vi "main.vi"() -> ()   [LabVIEW 2023] (continued)
  8        F0\t60\t22\tFC\tFF\tFF\tFF\t43\r\n      1144  0CF103A7   00000004    8        17\t1F\t08\t60\tB1\t1F\t08\t43\r\n      1144  0CF102A7   00000004    8        30\t75\tE0\t2E\t80\tFF\tFF\tFD\r\n      1143  0C3C4D4A   00000004    8        BE\tFF\tFF\t7F\t18\tFF\tFF\t43\r\n      1143  0CF101A7   00000004    8        68\t00\t97\tCC\t00\t15\t39\t53\r\n      1142  18F120F0   00000004    8        2B\t75\t60\tB1\tB0\t01\tFF\tFF\r\n      1141  18F11FF0   00000004    8        FF\t3F\t90\t68\t88\t1B\t10\t3C\r\n      1132  1FFFFFFF   00000004    8        00\t20\tFF\tFF\tFF\tFF\tFF\tFF\r\n      1147  18FEF117   00000004    8        F7\t97\tCC\tCF\tFF\tFF\tFF\tFF\r\n      1147  18F121F0   00000004    8        09\t18\t00\t00\tFF\tFF\tB0\t01\r\n      1146  18F108A7   00000004    8        F0\t00\t00\tFF\tFF\tFF\tFF\t40\r\n      1145  18F106A7   00000004    8        00\tF7\tFF\tFF\tFF\tFF\tFF\t87\r\n      1145  0CF104A7   00000004    8        F0\t60\t22\tFC\tFF\tFF\tFF\t43\r\n      1144  0CF103A7   00000004    8        17\t1F\t08\t60\tB1\t1F\t08\t43\r\n      1144  0CF102A7   00000004    8        30\t75\tE0\t2E\t80\tFF\tFF\tFD\r\n      1143  0C3C4D4A   00000004    8        BE\tFF\tFF\t7F\t18\tFF\tFF\t43\r\n      1143  0CF101A7   00000004    8        68\t00\t97\tCC\t00\t15\t39\t53\r\n      1142  18F120F0   00000004    8        2B\t75\t60\tB1\tB0\t01\tFF\tFF\r\n      1141  18F11FF0   00000004    8        FF\t3F\t90\t68\t88\t1B\t10\t3C\r\n      1148  1FFFFFFF   00000004    8        00\t00\tFF\tFF\tFF\tFF\tFF\tFF\r\n      1147  18FEF117   00000004    8        F7\t97\tCC\tCF\tFF\tFF\tFF\tFF\r\n      1147  18F121F0   00000004    8        09\t18\t00\t00\tFF\tFF\tB0\t01\r\n      1146  18F108A7   00000004    8        F0\t00\t00\tFF\tFF\tFF\tFF\t40\r\n      1145  18F106A7   00000004    8        00\tF7\tFF\tFF\tFF\tFF\tFF\t87\r\n      1145  0CF104A7   00000004    8        F0\t60\t22\tFC\tFF\tFF\tFF\t43\r\n      1144  0CF103A7   00000004    8        17\t1F\t08\t60\tB1\t1F\t08\t43\r\n      1144  0CF102A7   00000004    8        30\t75\tE0\t2E\t80\tFF\tFF\tFD\r\n      1143  0C3C4D4A   00000004    8        BE\tFF\tFF\t7F\t18\tFF\tFF\t43\r\n      1143  0CF101A7   00000004    8        68\t00\t97\tCC\t00\t15\t39\t53\r\n      1142  18F120F0   00000004    8        2B\t75\t60\tB1\tB0\t01\tFF\tFF\r\n      1152  1FFFFFFF   00000004    8        00\t20\tFF\tFF\tFF\tFF\tFF\tFF\r\n      1148  1FFFFFFF   00000004    8        00\t00\tFF\tFF\tFF\tFF\tFF\tFF\r\n      1147  18FEF117   00000004    8        F7\t97\tCC\tCF\tFF\tFF\tFF\tFF\r\n      1147  18F121F0   00000004    8        09\t18\t00\t00\tFF\tFF\tB0\t01\r\n      1146  18F108A7   00000004    8        F0\t00\t00\tFF\tFF\tFF\tFF\t40\r\n      1145  18F106A7   00000004    8        00\tF7\tFF\tFF\tFF\tFF\tFF\t87\r\n      1145  0CF104A7   00000004    8        F0\t60\t22\tFC\tFF\tFF\tFF\t43\r\n      1144  0CF103A7   00000004    8        17\t1F\t08\t60\tB1\t1F\t08\t43\r\n      1144  0CF102A7   00000004    8        30\t75\tE0\t2E\t80\tFF\tFF\tFD\r\n      1143  0C3C4D4A   00000004    8        BE\tFF\tFF\t7F\t18\tFF\tFF\t43\r\n      1143  0CF101A7   00000004    8        68\t00\t97\tCC\t00\t15\t39\t53\r\n      1162  1FFFFFFF   00000004    8        00\t20\tFF\tFF\tFF\tFF\tFF\tFF\r\n      1152  1FFFFFFF   00000004    8        00\t20\tFF\tFF\tFF\tFF\tFF\tFF\r\n      1148  1FFFFFFF   00000004    8        00\t00\tFF\tFF\tFF\tFF\tFF\tFF\r\n      1147  18FEF117   00000004    8        F7\t97\tCC\tCF\tFF\tFF\tFF\tFF\r\n      1147  18F121F0   00000004    8        09\t18\t00\t00\tFF\tFF\tB0\t01\r\n      1146  18F108A7   00000004    8        F0\t00\t00\tFF\tFF\tFF\tFF\t40\r\n      1145  18F106A7   00000004    8        00\tF7\tFF\tFF\tFF\tFF\tFF\t87\r\n      1145  0CF104A7   00000004    8        F0\t60\t22\tFC\tFF\tFF\tFF\t43\r\n      1144  0CF103A7   00000004    8        17\t1F\t08\t60\tB1\t1F\t08\t43\r\n      1144  0CF102A7   00000004    8        30\t75\tE0\t2E\t80\tFF\tFF\tFD\r\n      1143  0C3C4D4A   00000004    8        BE\tFF\tFF\t7F\t18\tFF\tFF\t43\r\n      1163  0CF101A7   00000004    8        68\t00\t97\tCC\t00\t15\t39\t54\r\n      1162  1FFFFFFF   00000004    8        00\t20\tFF\tFF\tFF\tFF\tFF\tFF\r\n      1152  1FFFFFFF   00000004    8        00\t20\tFF\tFF\tFF\tFF\tFF\tFF\r\n      1148  1FFFFFFF   00000004    8        00\t00\tFF\tFF\tFF\tFF\tFF\tFF\r\n      1147  18FEF117   00000004    8        F7\t97\tCC\tCF\tFF\tFF\tFF\tFF\r\n      1147  18F121F0   00000004    8        09\t18\t00\t00\tFF\tFF\tB0\t01\r\n      1146  18F108A7   00000004    8        F0\t00\t00\tFF\tFF\tFF\tFF\t40\r\n      1145  18F106A7   00000004    8        00\tF7\tFF\tFF\tFF\tFF\tFF\t87\r\n      1145  0CF104A7   00000004    8        F0\t60\t22\tFC\tFF\tFF\tFF\t43\r\n      1144  0CF103A7   00000004    8        17\t1F\t08\t60\tB1\t1F\t08\t43\r\n      1144  0CF102A7   00000004    8        30\t75\tE0\t2E\t80\tFF\tFF\tFD\r\n      1163  0CF102A7   00000004    8        30\t75\tE0\t2E\t80\tFF\tFF\tFD\r\n      1163  0CF101A7   00000004    8        68\t00\t97\tCC\t00\t15\t39\t54\r\n      1162  1FFFFFFF   00000004    8        00\t20\tFF\tFF\tFF\tFF\tFF\tFF\r\n      1152  1FFFFFFF   00000004    8        00\t20\tFF\tFF\tFF\tFF\tFF\tFF\r\n      1148  1FFFFFFF   00000004    8        00\t00\tFF\tFF\tFF\tFF\tFF\tFF\r\n      1147  18FEF117   00000004    8        F7\t97\tCC\tCF\tFF\tFF\tFF\tFF\r\n      1147  18F121F0   00000004    8        09\t18\t00\t00\tFF\tFF\tB0\t01\r\n      1146  18F108A7   00000004    8        F0\t00\t00\tFF\tFF\tFF\tFF\t40\r\n      1145  18F106A7   00000004    8        00\tF7\tFF\tFF\tFF\tFF\tFF\t87\r\n      1145  0CF104A7   00000004    8        F0\t60\t22\tFC\tFF\tFF\tFF\t43\r\n      1144  0CF103A7   00000004    8        17\t1F\t08\t60\tB1\t1F\t08\t43\r\n      1172  1FFFFFFF   00000004    8        00\t20\tFF\tFF\tFF\tFF\tFF\tFF\r\n      1163  0CF102A7   00000004    8        30\t75\tE0\t2E\t80\tFF\tFF\tFD\r\n      1163  0CF101A7   00000004    8        68\t00\t97\tCC\t00\t15\t39\t54\r\n      1162  1FFFFFFF   00000004    8        00\t20\tFF\tFF\tFF\tFF\tFF\tFF\r\n      1152  1FFFFFFF   00000004    8        00\t20\tFF\tFF\tFF\tFF\tFF\tFF\r\n      1148  1FFFFFFF   00000004    8        00\t00\tFF\tFF\tFF\tFF\tFF\tFF\r\n      1147  18FEF117   00000004    8        F7\t97\tCC\tCF\tFF\tFF\tFF\tFF\r\n      1147  18F121F0   00000004    8        09\t18\t00\t00\tFF\tFF\tB0\t01\r\n      1146  18F108A7   00000004    8        F0\t00\t00\tFF\tFF\tFF\tFF\t40\r\n      1145  18F106A7   00000004    8        00\tF7\tFF\tFF\tFF\tFF\tFF\t87\r\n      1145  0CF104A7   00000004    8        F0\t60\t22\tFC\tFF\tFF\tFF\t43\r\n      1182  1FFFFFFF   00000004    8        00\t00\tFF\tFF\tFF\tFF\tFF\tFF\r\n      1172  1FFFFFFF   00000004    8        00\t20\tFF\tFF\tFF\tFF\tFF\tFF\r\n      1163  0CF102A7   00000004    8        30\t75\tE0\t2E\t80\tFF\tFF\tFD\r\n      1163  0CF101A7   00000004    8        68\t00\t97\tCC\t00\t15\t39\t54\r\n      1162  1FFFFFFF   00000004    8        00\t20\tFF\tFF\tFF\tFF\tFF\tFF\r\n      1152  1FFFFFFF   00000004    8        00\t20\tFF\tFF\tFF\tFF\tFF\tFF\r\n      1148  1FFFFFFF   00000004    8        00\t00\tFF\tFF\tFF\tFF\tFF\tFF\r\n      1147  18FEF117   00000004    8        F7\t97\tCC\tCF\tFF\tFF\tFF\tFF\r\n      1147  18F121F0   00000004    8        09\t18\t00\t00\tFF\tFF\tB0\t01\r\n      1146  18F108A7   00000004    8        F0\t00\t00\tFF\tFF\tFF\tFF\t40\r\n      1145  18F106A7   00000004    8        00\tF7\tFF\tFF\tFF\tFF\tFF\t87\r\n      1183  0CF101A7   00000004    8        68\t00\t97\tCC\t00\t15\t39\t55\r\n      1182  1FFFFFFF   00000004    8        00\t00\tFF\tFF\tFF\tFF\tFF\tFF\r\n      1172  1FFFFFFF   00000004    8        00\t20\tFF\tFF\tFF\tFF\tFF\tFF\r\n      1163  0CF102A7   00000004    8        30\t75\tE0\t2E\t80\tFF\tFF\tFD\r\n      1163  0CF101A7   00000004    8        68\t00\t97\tCC\t00\t15\t39\t54\r\n      1162  1FFFFFFF   00000004    8        00\t20\tFF\tFF\tFF\tFF\tFF\tFF\r\n      1152  1FFFFFFF   00000004    8        00\t20\tFF\tFF\tFF\tFF\tFF\tFF\r\n      1148  1FFFFFFF   00000004    8        00\t00\tFF\tFF\tFF\tFF\tFF\tFF\r\n      1147  18FEF117   00000004    8        F7\t97\tCC\tCF\tFF\tFF\tFF\tFF\r\n      1147  18F121F0   00000004    8        09\t18\t00\t00\tFF\tFF\tB0\t01\r\n      1146  18F108A7   00000004    8        F0\t00\t00\tFF\tFF\tFF\tFF\t40\r\n      1183  0CF102A7   00000004    8        30\t75\tE0\t2E\t80\tFF\tFF\tFD\r\n      1183  0CF101A7   00000004    8        68\t00\t97\tCC\t00\t15\t39\t55\r\n      1182  1FFFFFFF   00000004    8        00\t00\tFF\tFF\tFF\tFF\tFF\tFF\r\n      1172  1FFFFFFF   00000004    8        00\t20\tFF\tFF\tFF\tFF\tFF\tFF\r\n      1163  0CF102A7   00000004    8        30\t75\tE0\t2E\t80\tFF\tFF\tFD\r\n      1163  0CF101A7   00000004    8        68\t00\t97\tCC\t00\t15\t39\t54\r\n      1162  1FFFFFFF   00000004    8        00\t20\tFF\tFF\tFF\tFF\tFF\tFF\r\n      1152  1FFFFFFF   00000004    8        00\t20\tFF\tFF\tFF\tFF\tFF\tFF\r\n      1148  1FFFFFFF   00000004    8        00\t00\tFF\tFF\tFF\tFF\tFF\tFF\r\n      1147  18FEF117   00000004    8        F7\t97\tCC\tCF\tFF\tFF\tFF\tFF\r\n      1147  18F121F0   00000004    8        09\t18\t00\t00\tFF\tFF\tB0\t01\r\n      1192  1FFFFFFF   00000004    8        00\t20\tFF\tFF\tFF\tFF\tFF\tFF\r\n      1183  0CF102A7   00000004    8        30\t75\tE0\t2E\t80\tFF\tFF\tFD\r\n      1183  0CF101A7   00000004    8        68\t00\t97\tCC\t00\t15\t39\t55\r\n      1182  1FFFFFFF   00000004    8        00\t00\tFF\tFF\tFF\tFF\tFF\tFF\r\n      1172  1FFFFFFF   00000004    8        00\t20\tFF\tFF\tFF\tFF\tFF\tFF\r\n      1163  0CF102A7   00000004    8        30\t75\tE0\t2E\t80\tFF\tFF\tFD\r\n      1163  0CF101A7   00000004    8        68\t00\t97\tCC\t00\t15\t39\t54\r\n      1162  1FFFFFFF   00000004    8        00\t20\tFF\tFF\tFF\tFF\tFF\tFF\r\n      1152  1FFFFFFF   00000004    8        00\t20\tFF\tFF\tFF\tFF\tFF\tFF\r\n      1148  1FFFFFFF   00000004    8        00\t00\tFF\tFF\tFF\tFF\tFF\tFF\r\n      1147  18FEF117   00000004    8        F7\t97\tCC\tCF\tFF\tFF\tFF\tFF\r\n      1193  18F106A7   00000004    8        00\tF7\tFF\tFF\tFF\tFF\tFF\t88\r\n      1192  1FFFFFFF   00000004    8        00\t20\tFF\tFF\tFF\tFF\tFF\tFF\r\n      1183  0CF102A7   00000004    8        30\t75\tE0\t2E\t80\tFF\tFF\tFD\r\n      1183  0CF101A7   00000004    8        68\t00\t97\tCC\t00\t15\t39\t55\r\n      1182  1FFFFFFF   00000004    8        00\t00\tFF\tFF\tFF\tFF\tFF\tFF\r\n      1172  1FFFFFFF   00000004    8        00\t20\tFF\tFF\tFF\tFF\tFF\tFF\r\n      1163  0CF102A7   00000004    8        30\t75\tE0\t2E\t80\tFF\tFF\tFD\r\n      1163  0CF101A7   00000004    8        68\t00\t97\tCC\t00\t15\t39\t54\r\n      1162  1FFFFFFF   00000004    8        00\t20\tFF\tFF\tFF\tFF\tFF\tFF\r\n      1152  1FFFFFFF   00000004    8        00\t20\tFF\tFF\tFF\tFF\tFF\tFF\r\n      1148  1FFFFFFF   00000004    8        00\t00\tFF\tFF\tFF\tFF\tFF\tFF\r\n      1202  1FFFFFFF   00000004    8        00\t00\tFF\tFF\tFF\tFF\tFF\tFF\r\n      1193  18F106A7   00000004    8        00\tF7\tFF\tFF\tFF\tFF\tFF\t88\r\n      1192  1FFFFFFF   00000004    8        00\t20\tFF\tFF\tFF\tFF\tFF\tFF\r\n      1183  0CF102A7   00000004    8        30\t75\tE0\t2E\t80\tFF\tFF\tFD\r\n      1183  0CF101A7   00000004    8        68\t00\t97\tCC\t00\t15\t39\t55\r\n      1182  1FFFFFFF   00000004    8        00\t00\tFF\tFF\tFF\tFF\tFF\tFF\r\n      1172  1FFFFFFF   00000004    8        00\t20\tFF\tFF\tFF\tFF\tFF\tFF\r\n      1163  0CF102A7   00000004    8        30\t75\tE0\t2E\t80\tFF\tFF\tFD\r\n      1163  0CF101A7   00000004    8        68\t00\t97\tCC\t00\t15\t39\t54\r\n      1162  1FFFFFFF   00000004    8        00\t20\tFF\tFF\tFF\tFF\tFF\tFF\r\n      1152  1FFFFFFF   00000004    8        00\t20\tFF\tFF\tFF\tFF\tFF\tFF\r\n      1203  0CF101A7   00000004    8        68\t00\t97\tCC\t00\t15\t39\t56\r\n      1202  1FFFFFFF   00000004    8        00\t00\tFF\tFF\tFF\tFF\tFF\tFF\r\n      1193  18F106A7   00000004    8        00\tF7\tFF\tFF\tFF\tFF\tFF\t88\r\n      1192  1FFFFFFF   00000004    8        00\t20\tFF\tFF\tFF\tFF\tFF\tFF\r\n      1183  0CF102A7   00000004    8        30\t75\tE0\t2E\t80\tFF\tFF\tFD\r\n      1183  0CF101A7   00000004    8        68\t00\t97\tCC\t00\t15\t39\t55\r\n      1182  1FFFFFFF   00000004    8        00\t00\tFF\tFF\tFF\tFF\tFF\tFF\r\n      1172  1FFFFFFF   00000004    8        00\t20\tFF\tFF\tFF\tFF\tFF\tFF\r\n      1163  0CF102A7   00000004    8        30\t75\tE0\t2E\t80\tFF\tFF\tFD\r\n      1163  0CF101A7   00000004    8        68\t00\t97\tCC\t00\t15\t39\t54\r\n      1162  1FFFFFFF   00000004    8        00\t20\tFF\tFF\tFF\tFF\tFF\tFF\r\n      1203  0CF102A7   00000004    8        30\t75\tE0\t2E\t80\tFF\tFF\tFD\r\n      1203  0CF101A7   00000004    8        68\t00\t97\tCC\t00\t15\t39\t56\r\n      1202  1FFFFFFF   00000004    8        00\t00\tFF\tFF\tFF\tFF\tFF\tFF\r\n      1193  18F106A7   00000004    8        00\tF7\tFF\tFF\tFF\tFF\tFF\t88\r\n      1192  1FFFFFFF   00000004    8        00\t20\tFF\tFF\tFF\tFF\tFF\tFF\r\n      1183  0CF102A7   00000004    8        30\t75\tE0\t2E\t80\tFF\tFF\tFD\r\n      1183  0CF101A7   00000004    8        68\t00\t97\tCC\t00\t15\t39\t55\r\n      1182  1FFFFFFF   00000004    8        00\t00\tFF\tFF\tFF\tFF\tFF\tFF\r\n      1172  1FFFFFFF   00000004    8        00\t20\tFF\tFF\tFF\tFF\tFF\tFF\r\n      1163  0CF102A7   00000004    8        30\t75\tE0\t2E\t80\tFF\tFF\tFD\r\n      1163  0CF101A7   00000004    8        68\t00\t97\tCC\t00\t15\t39\t54\r\n      1212  1FFFFFFF   00000004    8        00\t20\tFF\tFF\tFF\tFF\tFF\tFF\r\n      1203  0CF102A7   00000004    8        30\t75\tE0\t2E\t80\tFF\tFF\tFD\r\n      1203  0CF101A7   00000004    8        68\t00\t97\tCC\t00\t15\t39\t56\r\n      1202  1FFFFFFF   00000004    8        00\t00\tFF\tFF\tFF\tFF\tFF\tFF\r\n      1193  18F106A7   00000004    8        00\tF7\tFF\tFF\tFF\tFF\tFF\t88\r\n      1192  1FFFFFFF   00000004    8        00\t20\tFF\tFF\tFF\tFF\tFF\tFF\r\n      1183  0CF102A7   00000004    8        30\t75\tE0\t2E\t80\tFF\tFF\tFD\r\n      1183  0CF101A7   00000004    8        68\t00\t97\tCC\t00\t15\t39\t55\r\n      1182  1FFFFFFF   00000004    8        00\t00\tFF\tFF\tFF\tFF\tFF\tFF\r\n      1172  1FFFFFFF   00000004    8        00\t20\tFF\tFF\tFF\tFF\tFF\tFF\r\n      1163  0CF102A7   00000004    8        30\t75\tE0\t2E\t80\tFF\tFF\tFD\r\n      1222  1FFFFFFF   00000004    8        00\t00\tFF\tFF\tFF\tFF\tFF\tFF\r\n      1212  1FFFFFFF   00000004    8        00\t20\tFF\tFF\tFF\tFF\tFF\tFF\r\n      1203  0CF102A7   00000004    8        30\t75\tE0\t2E\t80\tFF\tFF\tFD\r\n      1203  0CF101A7   00000004    8        68\t00\t97\tCC\t00\t15\t39\t56\r\n      1202  1FFFFFFF   00000004    8        00\t00\tFF\tFF\tFF\tFF\tFF\tFF\r\n      1193  18F106A7   00000004    8        00\tF7\tFF\tFF\tFF\tFF\tFF\t88\r\n      1192  1FFFFFFF   00000004    8        00\t20\tFF\tFF\tFF\tFF\tFF\tFF\r\n      1183  0CF102A7   00000004    8        30\t75\tE0\t2E\t80\tFF\tFF\tFD\r\n      1183  0CF101A7   00000004    8        68\t00\t97\tCC\t00\t15\t39\t55\r\n      1182  1FFFFFFF   00000004    8        00\t00\tFF\tFF\tFF\tFF\tFF\tFF\r\n      1172  1FFFFFFF   00000004    8        00\t20\tFF\tFF\tFF\tFF\tFF\tFF\r\n      1223  0CF101A7   00000004    8        68\t00\t97\tCC\t00\t16\t39\t57\r\n      1222  1FFFFFFF   00000004    8        00\t00\tFF\tFF\tFF\tFF\tFF\tFF\r\n      1212  1FFFFFFF   00000004    8        00\t20\tFF\tFF\tFF\tFF\tFF\tFF\r\n      1203  0CF102A7   00000004    8        30\t75\tE0\t2E\t80\tFF\tFF\tFD\r\n      1203  0CF101A7   00000004    8        68\t00\t97\tCC\t00\t15\t39\t56\r\n      1202  1FFFFFFF   00000004    8        00\t00\tFF\tFF\tFF\tFF\tFF\tFF\r\n      1193  18F106A7   00000004    8        00\tF7\tFF\tFF\tFF\tFF\tFF\t88\r\n      1192  1FFFFFFF   00000004    8        00\t20\tFF\tFF\tFF\tFF\tFF\tFF\r\n      1183  0CF102A7   00000004    8        30\t75\tE0\t2E\t80\tFF\tFF\tFD\r\n      1183  0CF101A7   00000004    8        68\t00\t97\tCC\t00\t15\t39\t55\r\n      1182  1FFFFFFF   00000004    8        00\t00\tFF\tFF\tFF\tFF\tFF\tFF\r\n      1223  0CF102A7   00000004    8        30\t75\tE0\t2E\t80\tFF\tFF\tFD\r\n      1223  0CF101A7   00000004    8        68\t00\t97\tCC\t00\t16\t39\t57\r\n      1222  1FFFFFFF   00000004    8        00\t00\tFF\tFF\tFF\tFF\tFF\tFF\r\n      1212  1FFFFFFF   00000004    8        00\t20\tFF\tFF\tFF\tFF\tFF\tFF\r\n      1203  0CF102A7   00000004    8        30\t75\tE0\t2E\t80\tFF\tFF\tFD\r\n      1203  0CF101A7   00000004    8        68\t00\t97\tCC\t00\t15\t39\t56\r\n      1202  1FFFFFFF   00000004    8        00\t00\tFF\tFF\tFF\tFF\tFF\tFF\r\n      1193  18F106A7   00000004    8        00\tF7\tFF\tFF\tFF\tFF\tFF\t88\r\n      1192  1FFFFFFF   00000004    8        00\t20\tFF\tFF\tFF\tFF\tFF\tFF\r\n      1183  0CF102A7   00000004    8        30\t75\tE0\t2E\t80\tFF\tFF\tFD\r\n      1183  0CF101A7   00000004    8        68\t00\t97\tCC\t00\t15\t39\t55\r\n      1232  1FFFFFFF   00000004    8        00\t20\tFF\tFF\tFF\tFF\tFF\tFF\r\n      1223  0CF102A7   00000004    8        30\t75\tE0\t2E\t80\tFF\tFF\tFD\r\n      1223  0CF101A7   00000004    8        68\t00\t97\tCC\t00\t16\t39\t57\r\n      1222  1FFFFFFF   00000004    8        00\t00\tFF\tFF\tFF\tFF\tFF\tFF\r\n      1212  1FFFFFFF   00000004    8        00\t20\tFF\tFF\tFF\tFF\tFF\tFF\r\n      1203  0CF102A7   00000004    8        30\t75\tE0\t2E\t80\tFF\tFF\tFD\r\n      1203  0CF101A7   00000004    8        68\t00\t97\tCC\t00\t15\t39\t56\r\n      1202  1FFFFFFF   00000004    8        00\t00\tFF\tFF\tFF\tFF\tFF\tFF\r\n      1193  18F106A7   00000004    8        00\tF7\tFF\tFF\tFF\tFF\tFF\t88\r\n      1192  1FFFFFFF   00000004    8        00\t20\tFF\tFF\tFF\tFF\tFF\tFF\r\n      1183  0CF102A7   00000004    8        30\t75\tE0\t2E\t80\tFF\tFF\tFD\r\n      1241  18F11FF0   00000004    8        FF\t3F\t90\t68\t88\t1B\t10\t4C\r\n      1232  1FFFFFFF   00000004    8        00\t20\tFF\tFF\tFF\tFF\tFF\tFF\r\n      1223  0CF102A7   00000004    8        30\t75\tE0\t2E\t80\tFF\tFF\tFD\r\n      1223  0CF101A7   00000004    8        68\t00\t97\tCC\t00\t16\t39\t57\r\n      1222  1FFFFFFF   00000004    8        00\t00\tFF\tFF\tFF\tFF\tFF\tFF\r\n      1212  1FFFFFFF   00000004    8        00\t20\tFF\tFF\tFF\tFF\tFF\tFF\r\n      1203  0CF102A7   00000004    8        30\t75\tE0\t2E\t80\tFF\tFF\tFD\r\n      1203  0CF101A7   00000004    8        68\t00\t97\tCC\t00\t15\t39\t56\r\n      1202  1FFFFFFF   00000004    8        00\t00\tFF\tFF\tFF\tFF\tFF\tFF\r\n      1193  18F106A7   00000004    8        00\tF7\tFF\tFF\tFF\tFF\tFF\t88\r\n      1192  1FFFFFFF   00000004    8        00\t20\tFF\tFF\tFF\tFF\tFF\tFF\r\n      1242  18F120F0   00000004    8        2B\t75\t60\tB1\tB0\t01\tFF\tFF\r\n      1241  18F11FF0   00000004    8        FF\t3F\t90\t68\t88\t1B\t10\t4C\r\n      1232  1FFFFFFF   00000004    8        00\t20\tFF\tFF\tFF\tFF\tFF\tFF\r\n      1223  0CF102A7   00000004    8        30\t75\tE0\t2E\t80\tFF\tFF\tFD\r\n      1223  0CF101A7   00000004    8        68\t00\t97\tCC\t00\t16\t39\t57\r\n      1222  1FFFFFFF   00000004    8        00\t00\tFF\tFF\tFF\tFF\tFF\tFF\r\n      1212  1FFFFFFF   00000004    8        00\t20\tFF\tFF\tFF\tFF\tFF\tFF\r\n      1203  0CF102A7   00000004    8        30\t75\tE0\t2E\t80\tFF\tFF\tFD\r\n      1203  0CF101A7   00000004    8        68\t00\t97\tCC\t00\t15\t39\t56\r\n      1202  1FFFFFFF   00000004    8        00\t00\tFF\tFF\tFF\tFF\tFF\tFF\r\n      1193  18F106A7   00000004    8        00\tF7\tFF\tFF\tFF\tFF\tFF\t88\r\n      1243  0CF101A7   00000004    8        68\t00\t97\tCC\t00\t16\t39\t58\r\n      1242  18F120F0   00000004    8        2B\t75\t60\tB1\tB0\t01\tFF\tFF\r\n      1241  18F11FF0   00000004    8        FF\t3F\t90\t68\t88\t1B\t10\t4C\r\n      1232  1FFFFFFF   00000004    8        00\t20\tFF\tFF\tFF\tFF\tFF\tFF\r\n      1223  0CF102A7   00000004    8        30\t75\tE0\t2E\t80\tFF\tFF\tFD\r\n      1223  0CF101A7   00000004    8        68\t00\t97\tCC\t00\t16\t39\t57\r\n      1222  1FFFFFFF   00000004    8        00\t00\tFF\tFF\tFF\tFF\tFF\tFF\r\n      1212  1FFFFFFF   00000004    8        00\t20\tFF\tFF\tFF\tFF\tFF\tFF\r\n      1203  0CF102A7   00000004    8        30\t75\tE0\t2E\t80\tFF\tFF\tFD\r\n      1203  0CF101A7   00000004    8        68\t00\t97\tCC\t00\t15\t39\t56\r\n      1202  1FFFFFFF   00000004    8        00\t00\tFF\tFF\tFF\tFF\tFF\tFF\r\n      1243  0C3C4D4A   00000004    8        BE\tFF\tFF\t7F\t18\tFF\tFF\t44\r\n      1243  0CF101A7   00000004    8        68\t00\t97\tCC\t00\t16\t39\t58\r\n      1242  18F120F0   00000004    8        2B\t75\t60\tB1\tB0\t01\tFF\tFF\r\n      1241  18F11FF0   00000004    8        FF\t3F\t90\t68\t88\t1B\t10\t4C\r\n      1232  1FFFFFFF   00000004    8        00\t20\tFF\tFF\tFF\tFF\tFF\tFF\r\n      1223  0CF102A7   00000004    8        30\t75\tE0\t2E\t80\tFF\tFF\tFD\r\n      1223  0CF101A7   00000004    8        68\t00\t97\tCC\t00\t16\t39\t57\r\n      1222  1FFFFFFF   00000004    8        00\t00\tFF\tFF\tFF\tFF\tFF\tFF\r\n      1212  1FFFFFFF   00000004    8        00\t20\tFF\tFF\tFF\tFF\tFF\tFF\r\n      1203  0CF102A7   00000004    8        30\t75\tE0\t2E\t80\tFF\tFF\tFD\r\n      1203  0CF101A7   00000004    8        68\t00\t97\tCC\t00\t15\t39\t56\r\n      1244  0CF102A7   00000004    8        30\t75\tE0\t2E\t80\tFF\tFF\tFD\r\n      1243  0C3C4D4A   00000004    8        BE\tFF\tFF\t7F\t18\tFF\tFF\t44\r\n      1243  0CF101A7   00000004    8        68\t00\t97\tCC\t00\t16\t39\t58\r\n      1242  18F120F0   00000004    8        2B\t75\t60\tB1\tB0\t01\tFF\tFF\r\n      1241  18F11FF0   00000004    8        FF\t3F\t90\t68\t88\t1B\t10\t4C\r\n      1232  1FFFFFFF   00000004    8        00\t20\tFF\tFF\tFF\tFF\tFF\tFF\r\n      1223  0CF102A7   00000004    8        30\t75\tE0\t2E\t80\tFF\tFF\tFD\r\n      1223  0CF101A7   00000004    8        68\t00\t97\tCC\t00\t16\t39\t57\r\n      1222  1FFFFFFF   00000004    8        00\t00\tFF\tFF\tFF\tFF\tFF\tFF\r\n      1212  1FFFFFFF   00000004    8        00\t20\tFF\tFF\tFF\tFF\tFF\tFF\r\n      1203  0CF102A7   00000004    8        30\t75\tE0\t2E\t80\tFF\tFF\tFD\r\n      1244  0CF103A7   00000004    8        17\t1F\t08\t60\tB1\t1F\t08\t44\r\n      1244  0CF102A7   00000004    8        30\t75\tE0\t2E\t80\tFF\tFF\tFD\r\n      1243  0C3C4D4A   00000004    8        BE\tFF\tFF\t7F\t18\tFF\tFF\t44\r\n      1243  0CF101A7   00000004    8        68\t00\t97\tCC\t00\t16\t39\t58\r\n      1242  18F120F0   00000004    8        2B\t75\t60\tB1\tB0\t01\tFF\tFF\r\n      1241  18F11FF0   00000004    8        FF\t3F\t90\t68\t88\t1B\t10\t4C\r\n      1232  1FFFFFFF   00000004    8        00\t20\tFF\tFF\tFF\tFF\tFF\tFF\r\n      1223  0CF102A7   00000004    8        30\t75\tE0\t2E\t80\tFF\tFF\tFD\r\n      1223  0CF101A7   00000004    8        68\t00\t97\tCC\t00\t16\t39\t57\r\n      1222  1FFFFFFF   00000004    8        00\t00\tFF\tFF\tFF\tFF\tFF\tFF\r\n      1212  1FFFFFFF   00000004    8        00\t20\tFF\tFF\tFF\tFF\tFF\tFF\r\n      1245  0CF104A7   00000004    8        F0\t60\t22\tFC\tFF\tFF\tFF\t44\r\n      1244  0CF103A7   00000004    8        17\t1F\t08\t60\tB1\t1F\t08\t44\r\n      1244  0CF102A7   00000004    8        30\t75\tE0\t2E\t80\tFF\tFF\tFD\r\n      1243  0C3C4D4A   00000004    8        BE\tFF\tFF\t7F\t18\tFF\tFF\t44\r\n      1243  0CF101A7   00000004    8        68\t00\t97\tCC\t00\t16\t39\t58\r\n      1242  18F120F0   00000004    8        2B\t75\t60\tB1\tB0\t01\tFF\tFF\r\n      1241  18F11FF0   00000004    8        FF\t3F\t90\t68\t88\t1B\t10\t4C\r\n      1232  1FFFFFFF   00000004    8        00\t20\tFF\tFF\tFF\tFF\tFF\tFF\r\n      1223  0CF102A7   00000004    8        30\t75\tE0\t2E\t80\tFF\tFF\tFD\r\n      1223  0CF101A7   00000004    8        68\t00\t97\tCC\t00\t16\t39\t57\r\n      1222  1FFFFFFF   00000004    8        00\t00\tFF\tFF\tFF\tFF\tFF\tFF\r\n      1245  18F106A7   00000004    8        00\tF7\tFF\tFF\tFF\tFF\tFF\t89\r\n      1245  0CF104A7   00000004    8        F0\t60\t22\tFC\tFF\tFF\tFF\t44\r\n      1244  0CF103A7   00000004    8        17\t1F\t08\t60\tB1\t1F\t08\t44\r\n      1244  0CF102A7   00000004    8        30\t75\tE0\t2E\t80\tFF\tFF\tFD\r\n      1243  0C3C4D4A   00000004    8        BE\tFF\tFF\t7F\t18\tFF\tFF\t44\r\n      1243  0CF101A7   00000004    8        68\t00\t97\tCC\t00\t16\t39\t58\r\n      1242  18F120F0   00000004    8        2B\t75\t60\tB1\tB0\t01\tFF\tFF\r\n      1241  18F11FF0   00000004    8        FF\t3F\t90\t68\t88\t1B\t10\t4C\r\n      1232  1FFFFFFF   00000004    8        00\t20\tFF\tFF\tFF\tFF\tFF\tFF\r\n      1223  0CF102A7   00000004    8        30\t75\tE0\t2E\t80\tFF\tFF\tFD\r\n      1223  0CF101A7   00000004    8        68\t00\t97\tCC\t00\t16\t39\t57\r\n      1246  18F121F0   00000004    8        09\t18\t00\t00\tFF\tFF\tB0\t01\r\n      1245  18F106A7   00000004    8        00\tF7\tFF\tFF\tFF\tFF\tFF\t89\r\n      1245  0CF104A7   00000004    8        F0\t60\t22\tFC\tFF\tFF\tFF\t44\r\n      1244  0CF103A7   00000004    8        17\t1F\t08\t60\tB1\t1F\t08\t44\r\n      1244  0CF102A7   00000004    8        30\t75\tE0\t2E\t80\tFF\tFF\tFD\r\n      1243  0C3C4D4A   00000004    8        BE\tFF\tFF\t7F\t18\tFF\tFF\t44\r\n      1243  0CF101A7   00000004    8        68\t00\t97\tCC\t00\t16\t39\t58\r\n      1242  18F120F0   00000004    8        2B\t75\t60\tB1\tB0\t01\tFF\tFF\r\n      1241  18F11FF0   00000004    8        FF\t3F\t90\t68\t88\t1B\t10\t4C\r\n      1232  1FFFFFFF   00000004    8        00\t20\tFF\tFF\tFF\tFF\tFF\tFF\r\n      1223  0CF102A7   00000004    8        30\t75\tE0\t2E\t80\tFF\tFF\tFD\r\n      1247  1FFFFFFF   00000004    8        00\t20\tFF\tFF\tFF\tFF\tFF\tFF\r\n      1246  18F121F0   00000004    8        09\t18\t00\t00\tFF\tFF\tB0\t01\r\n      1245  18F106A7   00000004    8        00\tF7\tFF\tFF\tFF\tFF\tFF\t89\r\n      1245  0CF104A7   00000004    8        F0\t60\t22\tFC\tFF\tFF\tFF\t44\r\n      1244  0CF103A7   00000004    8        17\t1F\t08\t60\tB1\t1F\t08\t44\r\n      1244  0CF102A7   00000004    8        30\t75\tE0\t2E\t80\tFF\tFF\tFD\r\n      1243  0C3C4D4A   00000004    8        BE\tFF\tFF\t7F\t18\tFF\tFF\t44\r\n      1243  0CF101A7   00000004    8        68\t00\t97\tCC\t00\t16\t39\t58\r\n      1242  18F120F0   00000004    8        2B\t75\t60\tB1\tB0\t01\tFF\tFF\r\n      1241  18F11FF0   00000004    8        FF\t3F\t90\t68\t88\t1B\t10\t4C\r\n      1232  1FFFFFFF   00000004    8        00\t20\tFF\tFF\tFF\tFF\tFF\tFF\r\n      1252  1FFFFFFF   00000004    8        00\t20\tFF\tFF\tFF\tFF\tFF\tFF\r\n      1247  1FFFFFFF   00000004    8        00\t20\tFF\tFF\tFF\tFF\tFF\tFF\r\n      1246  18F121F0   00000004    8        09\t18\t00\t00\tFF\tFF\tB0\t01\r\n      1245  18F106A7   00000004    8        00\tF7\tFF\tFF\tFF\tFF\tFF\t89\r\n      1245  0CF104A7   00000004    8        F0\t60\t22\tFC\tFF\tFF\tFF\t44\r\n      1244  0CF103A7   00000004    8        17\t1F\t08\t60\tB1\t1F\t08\t44\r\n      1244  0CF102A7   00000004    8        30\t75\tE0\t2E\t80\tFF\tFF\tFD\r\n      1243  0C3C4D4A   00000004    8        BE\tFF\tFF\t7F\t18\tFF\tFF\t44\r\n      1243  0CF101A7   00000004    8        68\t00\t97\tCC\t00\t16\t39\t58\r\n      1242  18F120F0   00000004    8        2B\t75\t60\tB1\tB0\t01\tFF\tFF\r\n      1241  18F11FF0   00000004    8        FF\t3F\t90\t68\t88\t1B\t10\t4C\r\n      1262  1FFFFFFF   00000004    8        00\t00\tFF\tFF\tFF\tFF\tFF\tFF\r\n      1252  1FFFFFFF   00000004    8        00\t20\tFF\tFF\tFF\tFF\tFF\tFF\r\n      1247  1FFFFFFF   00000004    8        00\t20\tFF\tFF\tFF\tFF\tFF\tFF\r\n      1246  18F121F0   00000004    8        09\t18\t00\t00\tFF\tFF\tB0\t01\r\n      1245  18F106A7   00000004    8        00\tF7\tFF\tFF\tFF\tFF\tFF\t89\r\n      1245  0CF104A7   00000004    8        F0\t60\t22\tFC\tFF\tFF\tFF\t44\r\n      1244  0CF103A7   00000004    8        17\t1F\t08\t60\tB1\t1F\t08\t44\r\n      1244  0CF102A7   00000004    8        30\t75\tE0\t2E\t80\tFF\tFF\tFD\r\n      1243  0C3C4D4A   00000004    8        BE\tFF\tFF\t7F\t18\tFF\tFF\t44\r\n      1243  0CF101A7   00000004    8        68\t00\t97\tCC\t00\t16\t39\t58\r\n      1242  18F120F0   00000004    8        2B\t75\t60\tB1\tB0\t01\tFF\tFF\r\n      1263  0CF101A7   00000004    8        68\t00\t97\tCC\t00\t16\t39\t59\r\n      1262  1FFFFFFF   00000004    8        00\t00\tFF\tFF\tFF\tFF\tFF\tFF\r\n      1252  1FFFFFFF   00000004    8        00\t20\tFF\tFF\tFF\tFF\tFF\tFF\r\n      1247  1FFFFFFF   00000004    8        00\t20\tFF\tFF\tFF\tFF\tFF\tFF\r\n      1246  18F121F0   00000004    8        09\t18\t00\t00\tFF\tFF\tB0\t01\r\n      1245  18F106A7   00000004    8        00\tF7\tFF\tFF\tFF\tFF\tFF\t89\r\n      1245  0CF104A7   00000004    8        F0\t60\t22\tFC\tFF\tFF\tFF\t44\r\n      1244  0CF103A7   00000004    8        17\t1F\t08\t60\tB1\t1F\t08\t44\r\n      1244  0CF102A7   00000004    8        30\t75\tE0\t2E\t80\tFF\tFF\tFD\r\n      1243  0C3C4D4A   00000004    8        BE\tFF\tFF\t7F\t18\tFF\tFF\t44\r\n      1243  0CF101A7   00000004    8        68\t00\t97\tCC\t00\t16\t39\t58\r\n      1263  0CF102A7   00000004    8        30\t75\tE0\t2E\t80\tFF\tFF\tFD\r\n      1263  0CF101A7   00000004    8        68\t00\t97\tCC\t00\t16\t39\t59\r\n      1262  1FFFFFFF   00000004    8        00\t00\tFF\tFF\tFF\tFF\tFF\tFF\r\n      1252  1FFFFFFF   00000004    8        00\t20\tFF\tFF\tFF\tFF\tFF\tFF\r\n      1247  1FFFFFFF   00000004    8        00\t20\tFF\tFF\tFF\tFF\tFF\tFF\r\n      1246  18F121F0   00000004    8        09\t18\t00\t00\tFF\tFF\tB0\t01\r\n      1245  18F106A7   00000004    8        00\tF7\tFF\tFF\tFF\tFF\tFF\t89\r\n      1245  0CF104A7   00000004    8        F0\t60\t22\tFC\tFF\tFF\tFF\t44\r\n      1244  0CF103A7   00000004    8        17\t1F\t08\t60\tB1\t1F\t08\t44\r\n      1244  0CF102A7   00000004    8        30\t75\tE0\t2E\t80\tFF\tFF\tFD\r\n      1243  0C3C4D4A   00000004    8        BE\tFF\tFF\t7F\t18\tFF\tFF\t44\r\n      1272  1FFFFFFF   00000004    8        00\t20\tFF\tFF\tFF\tFF\tFF\tFF\r\n      1263  0CF102A7   00000004    8        30\t75\tE0\t2E\t80\tFF\tFF\tFD\r\n      1263  0CF101A7   00000004    8        68\t00\t97\tCC\t00\t16\t39\t59\r\n      1262  1FFFFFFF   00000004    8        00\t00\tFF\tFF\tFF\tFF\tFF\tFF\r\n      1252  1FFFFFFF   00000004    8        00\t20\tFF\tFF\tFF\tFF\tFF\tFF\r\n      1247  1FFFFFFF   00000004    8        00\t20\tFF\tFF\tFF\tFF\tFF\tFF\r\n      1246  18F121F0   00000004    8        09\t18\t00\t00\tFF\tFF\tB0\t01\r\n      1245  18F106A7   00000004    8        00\tF7\tFF\tFF\tFF\tFF\tFF\t89\r\n      1245  0CF104A7   00000004    8        F0\t60\t22\tFC\tFF\tFF\tFF\t44\r\n      1244  0CF103A7   00000004    8        17\t1F\t08\t60\tB1\t1F\t08\t44\r\n      1244  0CF102A7   00000004    8        30\t75\tE0\t2E\t80\tFF\tFF\tFD\r\n      1282  1FFFFFFF   00000004    8        00\t00\tFF\tFF\tFF\tFF\tFF\tFF\r\n      1272  1FFFFFFF   00000004    8        00\t20\tFF\tFF\tFF\tFF\tFF\tFF\r\n      1263  0CF102A7   00000004    8        30\t75\tE0\t2E\t80\tFF\tFF\tFD\r\n      1263  0CF101A7   00000004    8        68\t00\t97\tCC\t00\t16\t39\t59\r\n      1262  1FFFFFFF   00000004    8        00\t00\tFF\tFF\tFF\tFF\tFF\tFF\r\n      1252  1FFFFFFF   00000004    8        00\t20\tFF\tFF\tFF\tFF\tFF\tFF\r\n      1247  1FFFFFFF   00000004    8        00\t20\tFF\tFF\tFF\tFF\tFF\tFF\r\n      1246  18F121F0   00000004    8        09\t18\t00\t00\tFF\tFF\tB0\t01\r\n      1245  18F106A7   00000004    8        00\tF7\tFF\tFF\tFF\tFF\tFF\t89\r\n      1245  0CF104A7   00000004    8        F0\t60\t22\tFC\tFF\tFF\tFF\t44\r\n      1244  0CF103A7   00000004    8        17\t1F\t08\t60\tB1\t1F\t08\t44\r\n      1283  0CF101A7   00000004    8        68\t00\t97\tCC\t00\t16\t39\t5A\r\n      1282  1FFFFFFF   00000004    8        00\t00\tFF\tFF\tFF\tFF\tFF\tFF\r\n      1272  1FFFFFFF   00000004    8        00\t20\tFF\tFF\tFF\tFF\tFF\tFF\r\n      1263  0CF102A7   00000004    8        30\t75\tE0\t2E\t80\tFF\tFF\tFD\r\n      1263  0CF101A7   00000004    8        68\t00\t97\tCC\t00\t16\t39\t59\r\n      1262  1FFFFFFF   00000004    8        00\t00\tFF\tFF\tFF\tFF\tFF\tFF\r\n      1252  1FFFFFFF   00000004    8        00\t20\tFF\tFF\tFF\tFF\tFF\tFF\r\n      1247  1FFFFFFF   00000004    8        00\t20\tFF\tFF\tFF\tFF\tFF\tFF\r\n      1246  18F121F0   00000004    8        09\t18\t00\t00\tFF\tFF\tB0\t01\r\n      1245  18F106A7   00000004    8        00\tF7\tFF\tFF\tFF\tFF\tFF\t89\r\n      1245  0CF104A7   00000004    8        F0\t60\t22\tFC\tFF\tFF\tFF\t44\r\n      1283  0CF102A7   00000004    8        30\t75\tE0\t2E\t80\tFF\tFF\tFD\r\n      1283  0CF101A7   00000004    8        68\t00\t97\tCC\t00\t16\t39\t5A\r\n      1282  1FFFFFFF   00000004    8        00\t00\tFF\tFF\tFF\tFF\tFF\tFF\r\n      1272  1FFFFFFF   00000004    8        00\t20\tFF\tFF\tFF\tFF\tFF\tFF\r\n      1263  0CF102A7   00000004    8        30\t75\tE0\t2E\t80\tFF\tFF\tFD\r\n      1263  0CF101A7   00000004    8        68\t00\t97\tCC\t00\t16\t39\t59\r\n      1262  1FFFFFFF   00000004    8        00\t00\tFF\tFF\tFF\tFF\tFF\tFF\r\n      1252  1FFFFFFF   00000004    8        00\t20\tFF\tFF\tFF\tFF\tFF\tFF\r\n      1247  1FFFFFFF   00000004    8        00\t20\tFF\tFF\tFF\tFF\tFF\tFF\r\n      1246  18F121F0   00000004    8        09\t18\t00\t00\tFF\tFF\tB0\t01\r\n      1245  18F106A7   00000004    8        00\tF7\tFF\tFF\tFF\tFF\tFF\t89\r\n      1292  1FFFFFFF   00000004    8        00\t20\tFF\tFF\tFF\tFF\tFF\tFF\r\n      1283  0CF102A7   00000004    8        30\t75\tE0\t2E\t80\tFF\tFF\tFD\r\n      1283  0CF101A7   00000004    8        68\t00\t97\tCC\t00\t16\t39\t5A\r\n      1282  1FFFFFFF   00000004    8        00\t00\tFF\tFF\tFF\tFF\tFF\tFF\r\n      1272  1FFFFFFF   00000004    8        00\t20\tFF\tFF\tFF\tFF\tFF\tFF\r\n      1263  0CF102A7   00000004    8        30\t75\tE0\t2E\t80\tFF\tFF\tFD\r\n      1263  0CF101A7   00000004    8        68\t00\t97\tCC\t00\t16\t39\t59\r\n      1262  1FFFFFFF   00000004    8        00\t00\tFF\tFF\tFF\tFF\tFF\tFF\r\n      1252  1FFFFFFF   00000004    8        00\t20\tFF\tFF\tFF\tFF\tFF\tFF\r\n      1247  1FFFFFFF   00000004    8        00\t20\tFF\tFF\tFF\tFF\tFF\tFF\r\n      1246  18F121F0   00000004    8        09\t18\t00\t00\tFF\tFF\tB0\t01\r\n      1293  18F106A7   00000004    8        00\tF7\tFF\tFF\tFF\tFF\tFF\t8A\r\n      1292  1FFFFFFF   00000004    8        00\t20\tFF\tFF\tFF\tFF\tFF\tFF\r\n      1283  0CF102A7   00000004    8        30\t75\tE0\t2E\t80\tFF\tFF\tFD\r\n      1283  0CF101A7   00000004    8        68\t00\t97\tCC\t00\t16\t39\t5A\r\n      1282  1FFFFFFF   00000004    8        00\t00\tFF\tFF\tFF\tFF\tFF\tFF\r\n      1272  1FFFFFFF   00000004    8        00\t20\tFF\tFF\tFF\tFF\tFF\tFF\r\n      1263  0CF102A7   00000004    8        30\t75\tE0\t2E\t80\tFF\tFF\tFD\r\n      1263  0CF101A7   00000004    8        68\t00\t97\tCC\t00\t16\t39\t59\r\n      1262  1FFFFFFF   00000004    8        00\t00\tFF\tFF\tFF\tFF\tFF\tFF\r\n      1252  1FFFFFFF   00000004    8        00\t20\tFF\tFF\tFF\tFF\tFF\tFF\r\n      1247  1FFFFFFF   00000004    8        00\t20\tFF\tFF\tFF\tFF\tFF\tFF\r\n      1302  1FFFFFFF   00000004    8        00\t00\tFF\tFF\tFF\tFF\tFF\tFF\r\n      1293  18F106A7   00000004    8        00\tF7\tFF\tFF\tFF\tFF\tFF\t8A\r\n      1292  1FFFFFFF   00000004    8        00\t20\tFF\tFF\tFF\tFF\tFF\tFF\r\n      1283  0CF102A7   00000004    8        30\t75\tE0\t2E\t80\tFF\tFF\tFD\r\n      1283  0CF101A7   00000004    8        68\t00\t97\tCC\t00\t16\t39\t5A\r\n      1282  1FFFFFFF   00000004    8        00\t00\tFF\tFF\tFF\tFF\tFF\tFF\r\n      1272  1FFFFFFF   00000004    8        00\t20\tFF\tFF\tFF\tFF\tFF\tFF\r\n      1263  0CF102A7   00000004    8        30\t75\tE0\t2E\t80\tFF\tFF\tFD\r\n      1263  0CF101A7   00000004    8        68\t00\t97\tCC\t00\t16\t39\t59\r\n      1262  1FFFFFFF   00000004    8        00\t00\tFF\tFF\tFF\tFF\tFF\tFF\r\n      1252  1FFFFFFF   00000004    8        00\t20\tFF\tFF\tFF\tFF\tFF\tFF\r\n      1303  0CF101A7   00000004    8        68\t00\t97\tCC\t00\t16\t39\t5B\r\n      1302  1FFFFFFF   00000004    8        00\t00\tFF\tFF\tFF\tFF\tFF\tFF\r\n      1293  18F106A7   00000004    8        00\tF7\tFF\tFF\tFF\tFF\tFF\t8A\r\n      1292  1FFFFFFF   00000004    8        00\t20\tFF\tFF\tFF\tFF\tFF\tFF\r\n      1283  0CF102A7   00000004    8        30\t75\tE0\t2E\t80\tFF\tFF\tFD\r\n      1283  0CF101A7   00000004    8        68\t00\t97\tCC\t00\t16\t39\t5A\r\n      1282  1FFFFFFF   00000004    8        00\t00\tFF\tFF\tFF\tFF\tFF\tFF\r\n      1272  1FFFFFFF   00000004    8        00\t20\tFF\tFF\tFF\tFF\tFF\tFF\r\n      1263  0CF102A7   00000004    8        30\t75\tE0\t2E\t80\tFF\tFF\tFD\r\n      1263  0CF101A7   00000004    8        68\t00\t97\tCC\t00\t16\t39\t59\r\n      1262  1FFFFFFF   00000004    8        00\t00\tFF\tFF\tFF\tFF\tFF\tFF\r\n      1303  0CF102A7   00000004    8        30\t75\tE0\t2E\t80\tFF\tFF\tFD\r\n      1303  0CF101A7   00000004    8        68\t00\t97\tCC\t00\t16\t39\t5B\r\n      1302  1FFFFFFF   00000004    8        00\t00\tFF\tFF\tFF\tFF\tFF\tFF\r\n      1293  18F106A7   00000004    8        00\tF7\tFF\tFF\tFF\tFF\tFF\t8A\r\n      1292  1FFFFFFF   00000004    8        00\t20\tFF\tFF\tFF\tFF\tFF\tFF\r\n      1283  0CF102A7   00000004    8        30\t75\tE0\t2E\t80\tFF\tFF\tFD\r\n      1283  0CF101A7   00000004    8        68\t00\t97\tCC\t00\t16\t39\t5A\r\n      1282  1FFFFFFF   00000004    8        00\t00\tFF\tFF\tFF\tFF\tFF\tFF\r\n      1272  1FFFFFFF   00000004    8        00\t20\tFF\tFF\tFF\tFF\tFF\tFF\r\n      1263  0CF102A7   00000004    8        30\t75\tE0\t2E\t80\tFF\tFF\tFD\r\n      1263  0CF101A7   00000004    8        68\t00\t97\tCC\t00\t16\t39\t59\r\n      1312  1FFFFFFF   00000004    8        00\t20\tFF\tFF\tFF\tFF\tFF\tFF\r\n      1303  0CF102A7   00000004    8        30\t75\tE0\t2E\t80\tFF\tFF\tFD\r\n      1303  0CF101A7   00000004    8        68\t00\t97\tCC\t00\t16\t39\t5B\r\n      1302  1FFFFFFF   00000004    8        00\t00\tFF\tFF\tFF\tFF\tFF\tFF\r\n      1293  18F106A7   00000004    8        00\tF7\tFF\tFF\tFF\tFF\tFF\t8A\r\n      1292  1FFFFFFF   00000004    8        00\t20\tFF\tFF\tFF\tFF\tFF\tFF\r\n      1283  0CF102A7   00000004    8        30\t75\tE0\t2E\t80\tFF\tFF\tFD\r\n      1283  0CF101A7   00000004    8        68\t00\t97\tCC\t00\t16\t39\t5A\r\n      1282  1FFFFFFF   00000004    8        00\t00\tFF\tFF\tFF\tFF\tFF\tFF\r\n      1272  1FFFFFFF   00000004    8        00\t20\tFF\tFF\tFF\tFF\tFF\tFF\r\n      1263  0CF102A7   00000004    8        30\t75\tE0\t2E\t80\tFF\tFF\tFD\r\n      1322  1FFFFFFF   00000004    8        00\t00\tFF\tFF\tFF\tFF\tFF\tFF\r\n      1312  1FFFFFFF   00000004    8        00\t20\tFF\tFF\tFF\tFF\tFF\tFF\r\n      1303  0CF102A7   00000004    8        30\t75\tE0\t2E\t80\tFF\tFF\tFD\r\n      1303  0CF101A7   00000004    8        68\t00\t97\tCC\t00\t16\t39\t5B\r\n      1302  1FFFFFFF   00000004    8        00\t00\tFF\tFF\tFF\tFF\tFF\tFF\r\n      1293  18F106A7   00000004    8        00\tF7\tFF\tFF\tFF\tFF\tFF\t8A\r\n      1292  1FFFFFFF   00000004    8        00\t20\tFF\tFF\tFF\tFF\tFF\tFF\r\n      1283  0CF102A7   00000004    8        30\t75\tE0\t2E\t80\tFF\tFF\tFD\r\n      1283  0CF101A7   00000004    8        68\t00\t97\tCC\t00\t16\t39\t5A\r\n      1282  1FFFFFFF   00000004    8        00\t00\tFF\tFF\tFF\tFF\tFF\tFF\r\n      1272  1FFFFFFF   00000004    8        00\t20\tFF\tFF\tFF\tFF\tFF\tFF\r\n      1323  0CF101A7   00000004    8        68\t00\t97\tCC\t00\t16\t39\t5C\r\n      1322  1FFFFFFF   00000004    8        00\t00\tFF\tFF\tFF\tFF\tFF\tFF\r\n      1312  1FFFFFFF   00000004    8        00\t20\tFF\tFF\tFF\tFF\tFF\tFF\r\n      1303  0CF102A7   00000004    8        30\t75\tE0\t2E\t80\tFF\tFF\tFD\r\n      1303  0CF101A7   00000004    8        68\t00\t97\tCC\t00\t16\t39\t5B\r\n      1302  1FFFFFFF   00000004    8        00\t00\tFF\tFF\tFF\tFF\tFF\tFF\r\n      1293  18F106A7   00000004    8        00\tF7\tFF\tFF\tFF\tFF\tFF\t8A\r\n      1292  1FFFFFFF   00000004    8        00\t20\tFF\tFF\tFF\tFF\tFF\tFF\r\n      1283  0CF102A7   00000004    8        30\t75\tE0\t2E\t80\tFF\tFF\tFD\r\n      1283  0CF101A7   00000004    8        68\t00\t97\tCC\t00\t16\t39\t5A\r\n      1282  1FFFFFFF   
